vi "Main On Compile Action VI.vi"(8 "error in (no error)":errorcluster, 11 "Device Item Ref in":T1 format="%.0x") -> (0 "error out":errorcluster)   [LabVIEW 2013, in "Engine Simulation Toolkit System Explorer.lvlib"]
uses:
  Engine Simulation Toolkit System Explorer.lvlib
  <vilib>/NI Veristand/Custom Device API/Custom Device Item Ref.ctl
  Shared/Compiled Data.ctl
  Shared/Engine Init Data.ctl
  Shared/1.0 APU Engine Data.ctl
  Shared/1.0 APU Engine FIFO Idxs.ctl
  Shared/Engine Status Data.ctl
  Shared/1.0 Analog Replay Engine Data.ctl
  Shared/1.0 Analog Replay FIFO Idxs.ctl
  Shared/1.0 Digital Pattern Gen Engine Data.ctl
  Shared/1.0 Digital Pattern Gen FIFO Idxs.ctl
  Shared/1.0 Event Timing Capture Engine Data.ctl
  Shared/1.0 Event Timing Capture FIFO Idxs.ctl
  Shared/1.0 Event Timing Measure Engine Data.ctl
  Shared/1.0 Event Timing Measure FIFO Idxs.ctl
  Shared/1.0 Knock Sensor Engine Data.ctl
  Shared/1.0 Knock Sensor FIFO Idxs.ctl
  Shared/1.0 Knock Cylinder Engine Data.ctl
  Shared/1.0 Knock Cylinder FIFO Idxs.ctl
  Shared/1.0 Directional Speed Engine Data.ctl
  Shared/1.0 Directional Speed FIFO Idxs.ctl
  Shared/1.1 APU Engine Data.ctl
  Shared/1.1 Event Timing Measure Engine Data.ctl
  Shared/1.3 Digital Pattern Gen Engine Data.ctl
  Shared/1.3 Digital Pattern Gen FIFO Idxs.ctl
  Shared/Bitfile EST Version.ctl
  Shared/1.3 APU Engine Data.ctl
  Shared/Properties.vi
  <vilib>/NI Veristand/Custom Device API/Get Item Property (String).vi
  <vilib>/NI Veristand/Custom Device API/Set Item Property (Variant).vi
  <vilib>/NI Veristand/Custom Device API/Custom Device API.lvlib
  Shared/Engine Simulation Toolkit Shared.lvlib
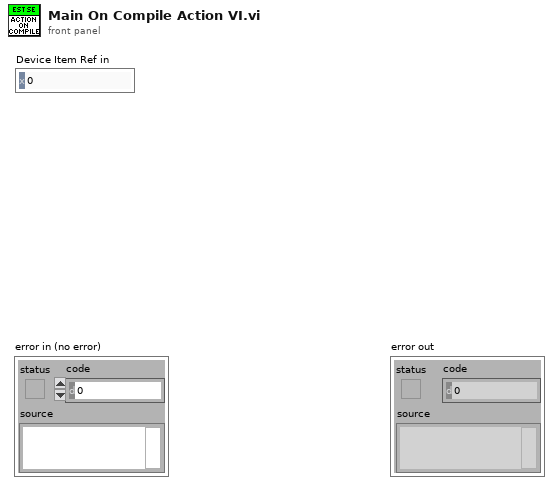
[diagram p1: front panel]
types:
  T1 = typedef "Custom Device API.lvlib/Custom Device Item Ref.ctl" = u64
  T2 = typedef "Engine Simulation Toolkit Shared.lvlib/Compiled Data.ctl" = cluster{"Init":T3, "1.0 APUs":T4[], "Status":T6, "DevOutFIFO":refnum<k33>, "DevInFIFO":refnum<k33>, "Device Inputs":dbl[], "Device Outputs":dbl[], "Last Device Inputs":dbl[], "1.0 Analog Replays":T7[], "Unused Analog Replays":string[], "1.0 Digital Pattern Gens":T9[], "Unused Digital Pattern Gens":string[], "1.0 Event Captures":T11[], "1.0 Event Measures":T13[], "1.0 Knock Sensors":T15[], "1.0 Knock Cylinders":T17[], "1.0 Directional Speed":T19[], "Unused Directional Sensors":string[], "1.1 APUs":T21[], "1.1 Event Measures":T22[], "1.3 Digital Pattern Gens":T23[], "Bitfile EST Version":T25, "1.3 APUs":T26[]}
  T3 = typedef "Engine Simulation Toolkit Shared.lvlib/Engine Init Data.ctl" = cluster{"CPU":i32, "RIO Address":string, "Decimation":i64, "Priority":i32, "Name":string, "Bitfile Path":path, "Input FIFO Size":i32, "Output FIFO Size":i32}
  T4 = typedef "Engine Simulation Toolkit Shared.lvlib/1.0 APU Engine Data.ctl" = cluster{"register names":cluster{"shared settings":string, "input":string, "settings":string, "output":string}, "shared settings":cluster{"cycle start":fxp<+,2,2>, "crank start":u16, "stuck limit":fxp<+,18,18>}, "settings":cluster{"acceleration":fxp<+,18,-20>, "max cycle":fxp<+,2,2>, "enable accel":bool}, "FIFO indexes":T5, "input":cluster{"desired speed":fxp<+/-,23,2>, "reset":bool}, "degrees of 1 cycle u16":dbl, "degrees of 1 crank u16":dbl}
  T5 = typedef "Engine Simulation Toolkit Shared.lvlib/1.0 APU Engine FIFO Idxs.ctl" = cluster{"inputs":cluster{"desired speed":i32, "reset":i32}, "outputs":cluster{"crank angle":i32, "cycle angle":i32, "actual speed":i32}}
  T6 = typedef "Engine Simulation Toolkit Shared.lvlib/Engine Status Data.ctl" = cluster{"FIFO indexes":cluster{"code":i32, "loop duration":i32, "late count":i32}}
  T7 = typedef "Engine Simulation Toolkit Shared.lvlib/1.0 Analog Replay Engine Data.ctl" = cluster{"register names":cluster{"load input":string, "settings":string, "input":string}, "settings":cluster{"ReverseNegate":bool, "CycleAngle":bool, "SpeedThreshold":fxp<+/-,23,2>, "AOBelowThreshold":i16}, "FIFO indexes":T8, "input":cluster{"Offset":i16, "VScaleSlope":fxp<+,18,6>, "VScaleIntercept":fxp<+/-,18,3>}, "offset convert":dbl, "DAC LUT":i16[], "SE_VScaleIntercept":fxp<+/-,18,3>, "SE_VScaleSlope":fxp<+,18,6>, "VOverride":bool, "ResetVolts":bool}
  T8 = typedef "Engine Simulation Toolkit Shared.lvlib/1.0 Analog Replay FIFO Idxs.ctl" = cluster{"enable voltage":i32, "volt slope":i32, "volt intercept":i32, "offset":i32}
  T9 = typedef "Engine Simulation Toolkit Shared.lvlib/1.0 Digital Pattern Gen Engine Data.ctl" = cluster{"register names":cluster{"load input":string, "settings":string, "input":string}, "settings":cluster{"edge 1":u16, "edge 2":u16, "cycle angle":bool, "enabled":bool, "first falling":bool}, "FIFO indexes":T10, "input":cluster{"Offset":i16}, "offset convert":dbl, "Position LUT":u16[]}
  T10 = typedef "Engine Simulation Toolkit Shared.lvlib/1.0 Digital Pattern Gen FIFO Idxs.ctl" = cluster{"offset":i32}
  T11 = typedef "Engine Simulation Toolkit Shared.lvlib/1.0 Event Timing Capture Engine Data.ctl" = cluster{"register names":cluster{"output":string}, "FIFO indexes":T12, "degrees of 1 u16":dbl, "wrap":bool, "window min":u16, "duration convert":dbl, "default start":dbl, "default end":dbl, "ref angle":dbl}
  T12 = typedef "Engine Simulation Toolkit Shared.lvlib/1.0 Event Timing Capture FIFO Idxs.ctl" = cluster{"start angle":i32, "end angle":i32, "duration":i32}
  T13 = typedef "Engine Simulation Toolkit Shared.lvlib/1.0 Event Timing Measure Engine Data.ctl" = cluster{"register names":cluster{"settings":string, "output":string}, "settings":cluster{"max":u16, "min":u16, "active high":bool, "wrap":bool, "full window":bool}, "FIFO indexes":T14}
  T14 = typedef "Engine Simulation Toolkit Shared.lvlib/1.0 Event Timing Measure FIFO Idxs.ctl" = cluster{"stuck active":i32, "win all active":i32, "win orph start":i32, "win orph end":i32}
  T15 = typedef "Engine Simulation Toolkit Shared.lvlib/1.0 Knock Sensor Engine Data.ctl" = cluster{"register names":cluster{"settings":string, "input":string}, "settings":cluster{"low freq (periods/tick)":fxp<+,32,0>, "high freq (periods/tick)":fxp<+,32,0>, "duration (1.25MHz tics)":fxp<+,18,18>, "low freq speed slope":fxp<+,16,-3>, "low freq speed intercept":fxp<+,10,-10>, "low freq by speed":bool}, "DAC multiplier":dbl, "FIFO indexes":T16, "input":cluster{"low freq scaler":fxp<+,10,0>}}
  T16 = typedef "Engine Simulation Toolkit Shared.lvlib/1.0 Knock Sensor FIFO Idxs.ctl" = cluster{"amp":i32}
  T17 = typedef "Engine Simulation Toolkit Shared.lvlib/1.0 Knock Cylinder Engine Data.ctl" = cluster{"register names":cluster{"settings":string, "input":string}, "settings":cluster{"seed":u16, "reset":bool}, "input":cluster{"probability compare":u16, "high freq scaler":fxp<+,10,0>, "trigger position":u16}, "DAC multiplier":dbl, "FIFO indexes":T18, "Angle multiplier":dbl}
  T18 = typedef "Engine Simulation Toolkit Shared.lvlib/1.0 Knock Cylinder FIFO Idxs.ctl" = cluster{"prob":i32, "amp":i32, "pos":i32}
  T19 = typedef "Engine Simulation Toolkit Shared.lvlib/1.0 Directional Speed Engine Data.ctl" = cluster{"register names":cluster{"settings":string, "input":string, "load input":string}, "settings":cluster{"Upper Value":u16, "Lower Value":u16, "Upper Index":fxp<+,10,10>, "Lower Index":fxp<+,10,10>, "Enabled":bool}, "input":cluster{"td (tics)":u16, "tf (tics)":u16, "tr (tics)":u16}, "FIFO indexes":T20, "Tooth Centers LUT":u16[]}
  T20 = typedef "Engine Simulation Toolkit Shared.lvlib/1.0 Directional Speed FIFO Idxs.ctl" = cluster{"td":i32, "tf":i32, "tr":i32}
  T21 = typedef "Engine Simulation Toolkit Shared.lvlib/1.1 APU Engine Data.ctl" = cluster{"register names":cluster{"shared settings":string, "input":string, "settings":string, "output":string, "go":string}, "shared settings":cluster{"cycle start":fxp<+,2,2>, "crank start":u16, "stuck limit":fxp<+,18,18>}, "settings":cluster{"acceleration":fxp<+,18,-20>, "max cycle":fxp<+,2,2>, "enable accel":bool}, "FIFO indexes":T5, "input":cluster{"desired speed":fxp<+/-,23,2>, "reset":bool}, "degrees of 1 cycle u16":dbl, "degrees of 1 crank u16":dbl}
  T22 = typedef "Engine Simulation Toolkit Shared.lvlib/1.1 Event Timing Measure Engine Data.ctl" = cluster{"register names":cluster{"settings":string, "output":string}, "settings":cluster{"max":u16, "min":u16, "active high":bool, "wrap":bool}, "FIFO indexes":T14}
  T23 = typedef "Engine Simulation Toolkit Shared.lvlib/1.3 Digital Pattern Gen Engine Data.ctl" = cluster{"register names":cluster{"load input":string, "settings":string, "input":string}, "settings":cluster{"edge 1":u16, "edge 2":u16, "cycle angle":bool, "enabled":bool, "first falling":bool, "fault":bool, "fault wrap":bool, "fault value":bool, "fault count":fxp<+,4,4>, "use fault count":bool}, "FIFO indexes":T24, "input":cluster{"Offset":i16}, "deg to u16 scale":dbl, "Position LUT":u16[], "# of teeth":i16, "max angle":dbl}
  T24 = typedef "Engine Simulation Toolkit Shared.lvlib/1.3 Digital Pattern Gen FIFO Idxs.ctl" = cluster{"offset":i32, "command":i32, "rotations":i32, "start angle":i32, "stop angle":i32, "tooth to rem":i32, "trigger":i32, "valid":i32}
  T25 = typedef "Engine Simulation Toolkit Shared.lvlib/Bitfile EST Version.ctl" = enum16{"1.0", "1.1", "1.2", "1.3"}
  T26 = typedef "Engine Simulation Toolkit Shared.lvlib/1.3 APU Engine Data.ctl" = cluster{"register names":cluster{"shared settings":string, "input":string, "settings":string, "output":string, "go":string}, "shared settings":cluster{"start":fxp<+,17,17>, "stuck limit":fxp<+,18,18>}, "settings":cluster{"acceleration":fxp<+,18,-20>, "enable accel":bool}, "FIFO indexes":T5, "input":cluster{"desired speed":fxp<+/-,23,2>, "reset":bool}, "degrees of 1 cycle u16":dbl, "degrees of 1 crank u16":dbl}
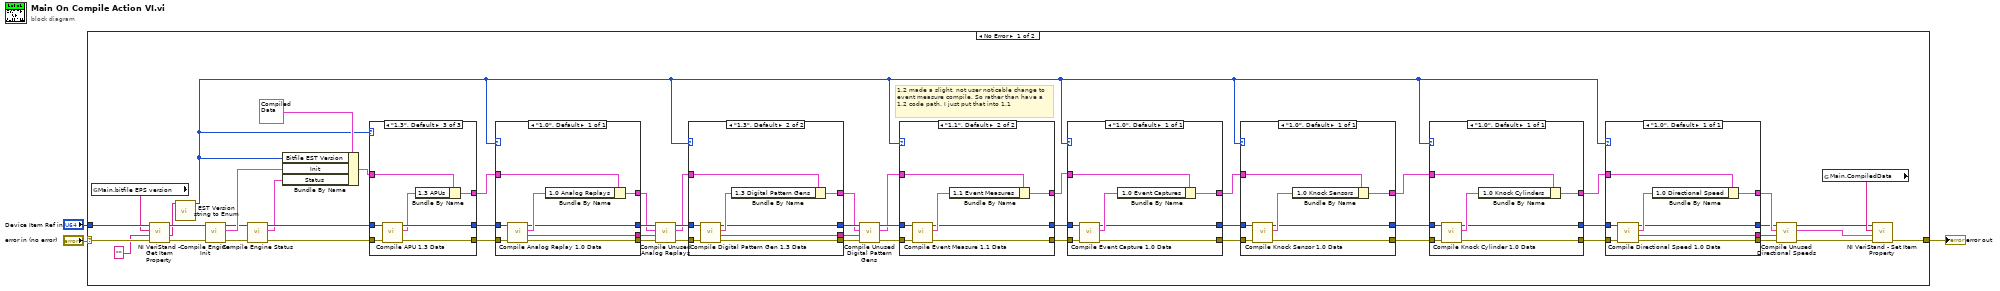
[diagram p0: block diagram]
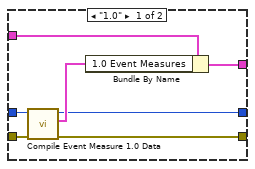
[diagram p2: hidden frame]
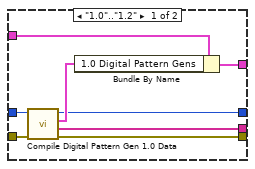
[diagram p3: hidden frame]
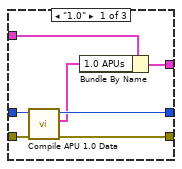
[diagram p4: hidden frame]
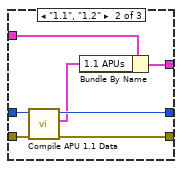
[diagram p5: hidden frame]
diagram:
  n1 = case shown="No Error" "error in (no error)" {
    selector: "error in (no error)" -> [w51 w146]
    tunnel: [w57 w146] -> w2
    tunnel: "Device Item Ref in" -> [w48 _]
    frame No Error {
      # "1.2 made a slight, not user noticable change to event measure compile. So rather than have a 1.2 code path, I just put that into 1.1"
      n2 = global read "Properties.vi" "Main.bitfile EPS version"() -> (w47:string)
      n3 = call-poly <vilib>:"NI VeriStand - Get Item Property.vi"("error in (no error)"=w51, "Default Value"="", "Property Name"=w47, "Item Ref in"=w48) -> ("error out"=w50:errorcluster, "Value"=w15:string, "Item Ref out"=w49:T1)  [unwired: 4 in, 1 out]
      n4 = call "EST Version string to Enum.vi"("EST version string"=w15) -> ("EST version enum"=w4:T25)  [unwired: 9 in, 1 out]
      n5 = call "Compile Engine Init.vi"("error in (no error)"=w50, "Device Item Ref in"=w49) -> ("error out"=w54:errorcluster, "System"=w53:T3, "Device Item Ref out"=w38:T1)  [unwired: 7 in]
      n6 = call "Compile Engine Status.vi"("error in (no error)"=w54, "Device Item Ref in"=w38) -> ("error out"=w39:errorcluster, "Status"=w36:T6, "Device Item Ref out"=w37:T1)  [unwired: 7 in]
      n7 = Bundle By Name(cluster=T2 {"Init"={"CPU"=0, "RIO Address"="", "Decimation"=0, "Priority"=0, "Name"="", "Bitfile Path"=path "", "Input FIFO Size"=0, "Output FIFO Size"=0}, "1.0 APUs"=[], "Status"={"FIFO indexes"={"code"=0, "loop duration"=0, "late count"=0}}, "DevOutFIFO"=refnum, "DevInFIFO"=refnum, "Device Inputs"=[], "Device Outputs"=[], "Last Device Inputs"=[], "1.0 Analog Replays"=[], "Unused Analog Replays"=[], "1.0 Digital Pattern Gens"=[], "Unused Digital Pattern Gens"=[], "1.0 Event Captures"=[], "1.0 Event Measures"=[], "1.0 Knock Sensors"=[], "1.0 Knock Cylinders"=[], "1.0 Directional Speed"=[], "Unused Directional Sensors"=[], "1.1 APUs"=[], "1.1 Event Measures"=[], "1.3 Digital Pattern Gens"=[], "Bitfile EST Version"=enum."1.0", "1.3 APUs"=[]} ("Compiled Data"), "Bitfile EST Version"=w4, "Init"=w53, "Status"=w36) -> (w52:T2)
      n8 = case shown="\"1.3\", Default" w4 {
        tunnel: w39 -> [w131 w138 w145]
        tunnel: [w130 w137 w144] -> w45
        tunnel: w37 -> [w129 w136 w143]
        tunnel: [w128 w135 w142] -> w44
        tunnel: w52 -> [w127 w134 w141]
        tunnel: [w125 w133 w140] -> w46
        frame "1.0" {
          n9 = call "Compile APU 1.0 Data.vi"("error in (no error)"=w131, "Device Item Ref in"=w129) -> ("error out"=w130:errorcluster, "APUs"=w126:T4[], "Device Item Ref out"=w128:T1)  [unwired: 7 in]
          n10 = Bundle By Name(cluster=w127, "1.0 APUs"=w126) -> (w125:T2)
        }
        frame "1.1", "1.2" {
          n11 = call "Compile APU 1.1 Data.vi"("error in (no error)"=w138, "Device Item Ref in"=w136) -> ("error out"=w137:errorcluster, "APUs"=w132:T21[], "Device Item Ref out"=w135:T1)  [unwired: 7 in]
          n12 = Bundle By Name(cluster=w134, "1.1 APUs"=w132) -> (w133:T2)
        }
        frame "1.3", Default {
          n13 = call "Compile APU 1.3 Data.vi"("error in (no error)"=w145, "Device Item Ref in"=w143) -> ("error out"=w144:errorcluster, "APUs"=w139:T26[], "Device Item Ref out"=w142:T1)  [unwired: 7 in]
          n14 = Bundle By Name(cluster=w141, "1.3 APUs"=w139) -> (w140:T2)
        }
      }
      n15 = case shown="\"1.0\", Default" w4 {
        tunnel: [w119] -> w43
        tunnel: w44 -> [w124]
        tunnel: [w118] -> w42
        tunnel: w46 -> [w123]
        tunnel: [w121] -> w41
        tunnel: w45 -> [w120]
        tunnel: [w117] -> w40
        frame "1.0", Default {
          n16 = call "Compile Analog Replay 1.0 Data.vi"("error in (no error)"=w120, "Device Item Ref in"=w124) -> ("error out"=w119:errorcluster, "bitfile names"=w117:string[], "Analog Replays"=w122:T7[], "Device Item Ref out"=w118:T1)  [unwired: 6 in]
          n17 = Bundle By Name(cluster=w123, "1.0 Analog Replays"=w122) -> (w121:T2)
        }
      }
      n18 = call "Compile Unused Analog Replays.vi"("error in (no error)"=w43, "bitfile names"=w40, "Compiled Data in"=w41, "Device Item Ref in"=w42) -> ("error out"=w34:errorcluster, "Compiled Data out"=w33:T2, "Item Ref out"=w35:T1)  [unwired: 5 in]
      n19 = case shown="\"1.3\", Default" w4 {
        tunnel: [w103 w111] -> w32
        tunnel: w35 -> [w108 w116]
        tunnel: [w102 w110] -> w30
        tunnel: w33 -> [w107 w115]
        tunnel: [w105 w113] -> w29
        tunnel: w34 -> [w104 w112]
        tunnel: [w101 w109] -> w31
        frame "1.0".."1.2" {
          n20 = call "Compile Digital Pattern Gen 1.0 Data.vi"("error in (no error)"=w104, "Device Item Ref in"=w108) -> ("error out"=w103:errorcluster, "bitfile names"=w101:string[], "Digital Pattern Gens"=w106:T9[], "Device Item Ref out"=w102:T1)  [unwired: 6 in]
          n21 = Bundle By Name(cluster=w107, "1.0 Digital Pattern Gens"=w106) -> (w105:T2)
        }
        frame "1.3", Default {
          n22 = call "Compile Digital Pattern Gen 1.3 Data.vi"("error in (no error)"=w112, "Device Item Ref in"=w116) -> ("error out"=w111:errorcluster, "bitfile names"=w109:string[], "Digital Pattern Gens"=w114:T23[], "Device Item Ref out"=w110:T1)  [unwired: 6 in]
          n23 = Bundle By Name(cluster=w115, "1.3 Digital Pattern Gens"=w114) -> (w113:T2)
        }
      }
      n24 = call "Compile Unused Digital Pattern Gens.vi"("error in (no error)"=w32, "bitfile names"=w31, "Compiled Data in"=w29, "Device Item Ref in"=w30) -> ("error out"=w28:errorcluster, "Compiled Data out"=w26:T2, "Item Ref out"=w27:T1)  [unwired: 5 in]
      n25 = case shown="\"1.1\", Default" w4 {
        tunnel: [w88 w95] -> w23
        tunnel: w27 -> [w93 w100]
        tunnel: [w87 w94] -> w25
        tunnel: w26 -> [w92 w99]
        tunnel: [w90 w97] -> w24
        tunnel: w28 -> [w89 w96]
        frame "1.0" {
          n26 = call "Compile Event Measure 1.0 Data.vi"("error in (no error)"=w89, "Device Item Ref in"=w93) -> ("error out"=w88:errorcluster, "Event Timing Measures"=w91:T13[], "Device Item Ref out"=w87:T1)  [unwired: 7 in]
          n27 = Bundle By Name(cluster=w92, "1.0 Event Measures"=w91) -> (w90:T2)
        }
        frame "1.1", Default {
          n28 = call "Compile Event Measure 1.1 Data.vi"("error in (no error)"=w96, "Device Item Ref in"=w100) -> ("error out"=w95:errorcluster, "Event Timing Measures"=w98:T22[], "Device Item Ref out"=w94:T1)  [unwired: 7 in]
          n29 = Bundle By Name(cluster=w99, "1.1 Event Measures"=w98) -> (w97:T2)
        }
      }
      n30 = case shown="\"1.0\", Default" w4 {
        tunnel: [w81] -> w20
        tunnel: w25 -> [w86]
        tunnel: [w80] -> w21
        tunnel: w24 -> [w85]
        tunnel: [w83] -> w22
        tunnel: w23 -> [w82]
        frame "1.0", Default {
          n31 = call "Compile Event Capture 1.0 Data.vi"("error in (no error)"=w82, "Device Item Ref in"=w86) -> ("error out"=w81:errorcluster, "Event Timing Captures"=w84:T11[], "Device Item Ref out"=w80:T1)  [unwired: 7 in]
          n32 = Bundle By Name(cluster=w85, "1.0 Event Captures"=w84) -> (w83:T2)
        }
      }
      n33 = case shown="\"1.0\", Default" w4 {
        tunnel: [w74] -> w18
        tunnel: w21 -> [w79]
        tunnel: [w73] -> w19
        tunnel: w22 -> [w78]
        tunnel: [w76] -> w17
        tunnel: w20 -> [w75]
        frame "1.0", Default {
          n34 = call "Compile Knock Sensor 1.0 Data.vi"("error in (no error)"=w75, "Device Item Ref in"=w79) -> ("error out"=w74:errorcluster, "Knock Sensors"=w77:T15[], "Device Item Ref out"=w73:T1)  [unwired: 7 in]
          n35 = Bundle By Name(cluster=w78, "1.0 Knock Sensors"=w77) -> (w76:T2)
        }
      }
      n36 = case shown="\"1.0\", Default" w4 {
        tunnel: [w67] -> w9
        tunnel: w19 -> [w72]
        tunnel: [w66] -> w8
        tunnel: w17 -> [w71]
        tunnel: [w69] -> w10
        tunnel: w18 -> [w68]
        frame "1.0", Default {
          n37 = call "Compile Knock Cylinder 1.0 Data.vi"("error in (no error)"=w68, "Device Item Ref in"=w72) -> ("error out"=w67:errorcluster, "Knock Cylinders"=w70:T17[], "Device Item Ref out"=w66:T1)  [unwired: 7 in]
          n38 = Bundle By Name(cluster=w71, "1.0 Knock Cylinders"=w70) -> (w69:T2)
        }
      }
      n39 = case shown="\"1.0\", Default" w4 {
        tunnel: [w60] -> w11
        tunnel: w8 -> [w65]
        tunnel: [w59] -> w13
        tunnel: w10 -> [w64]
        tunnel: [w62] -> w14
        tunnel: w9 -> [w61]
        tunnel: [w58] -> w12
        frame "1.0", Default {
          n40 = call "Compile Directional Speed 1.0 Data.vi"("error in (no error)"=w61, "Device Item Ref in"=w65) -> ("error out"=w60:errorcluster, "bitfile names"=w58:string[], "Directional Speeds"=w63:T19[], "Device Item Ref out"=w59:T1)  [unwired: 6 in]
          n41 = Bundle By Name(cluster=w64, "1.0 Directional Speed"=w63) -> (w62:T2)
        }
      }
      n42 = call "Compile Unused Directional Speeds.vi"("error in (no error)"=w11, "bitfile names"=w12, "Compiled Data in"=w14, "Device Item Ref in"=w13) -> ("error out"=w6:errorcluster, "Compiled Data out"=w5:T2, "Item Ref out"=w7:T1)  [unwired: 5 in]
      n43 = global read "Properties.vi" "Main.CompiledData"() -> (w56:string)
      n44 = call-poly <vilib>:"NI VeriStand - Set Item Property.vi"("error in (no error)"=w6, "Value"=w5, "Property Name"=w56, "Item Ref in"=w7) -> ("error out"=w57:errorcluster)  [unwired: 5 in, 2 out]
    }
    frame Error {
    }
  }
  "error out" <- w2
